vi "find_AnalysisObject_by_SessionID.vi"(8 "error in (no error)":errorcluster, 10 "SessionID":string, 11 "AnalysisObjects in":refnum<class "Analysis.lvclass">[](array[class])) -> (0 "error out":errorcluster, 1 "index of found":i32, 2 "found AnalyisObject":refnum<class "Analysis.lvclass">, 3 "AnalysisObjects out":refnum<class "Analysis.lvclass">[](array[class]))   [LabVIEW 2017]
doc: "Find the correct AnalysisObject by the SessionID"
uses:
  Classes/Analysis/Analysis.lvclass
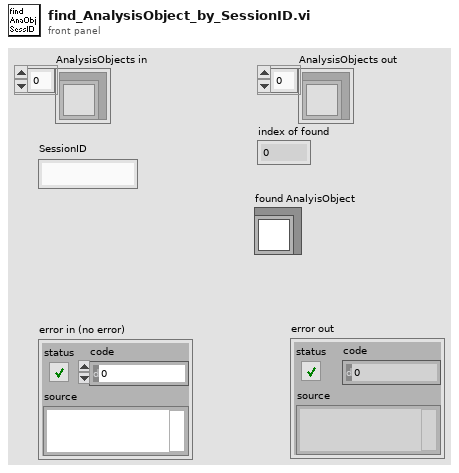
[diagram p1: front panel]
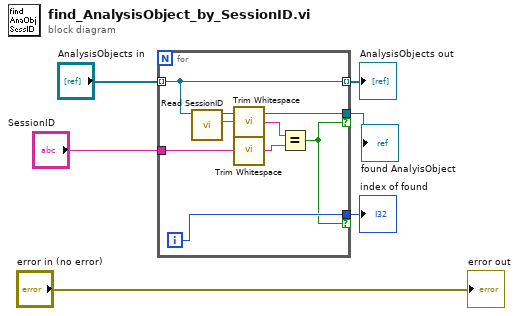
[diagram p0: block diagram]
diagram:
  n1 = for {
    tunnel: "AnalysisObjects in" -> [w9] mode=indexing
    tunnel: "SessionID" -> [w13]
    tunnel: [w10] -> w2 if=w7
    tunnel: [w9] -> w4 mode=indexing
    tunnel: [w8] -> w3 if=w7
    i -> [w8]
    n2 = call-dynamic "Read SessionID.vi"("Analysis in"=w9) -> ("SessionID"=w14:string, "Analysis out"=w10:refnum<class "Analysis.lvclass">)  [unwired: 8 in, 1 out]
    n3 = call <vilib>:"Trim Whitespace.vi"("string"=w14) -> ("trimmed string"=w12:string)  [unwired: 1 in]
    n4 = call <vilib>:"Trim Whitespace.vi"("string"=w13) -> ("trimmed string"=w11:string)  [unwired: 1 in]
    n5 = Equal?(x=w12, y=w11) -> (x = y?=w7:bool)
  }
  "found AnalyisObject" <- w2
  "AnalysisObjects out" <- w4
  "index of found" <- w3
  "error out" <- "error in (no error)"
